vi "LibXML_AddNextSibling.vi"(8 "error in":errorcluster, 10 "sibling node":u32, 11 "new node":u32) -> (0 "error out":errorcluster, 3 "node copy":u32)   [LabVIEW 2019, in "Tools.lvlib" / "LibXML.lvlib"]
doc: "libXML2:\nFunction: xmlAddNextSibling\n\nxmlNodePtr xmlAddNextSibling (xmlNodePtr cur, xmlNodePtr elem)\n\n\nAdd a new node @elem as the next sibling of @cur If the new node was already inserted in \na document it is first unlinked from its existing context. As a result of text merging @elem\nmay be freed. If the new node is ATTRIBUTE, it is added into properties instead of children. \nIf there is an attribute with equal name, it is first destroyed.\n\nparent: the parent node\ncur: the child node\nReturns: the child or NULL in case of error."
uses:
  LibXML.lvlib
  dll/libxml2.dll
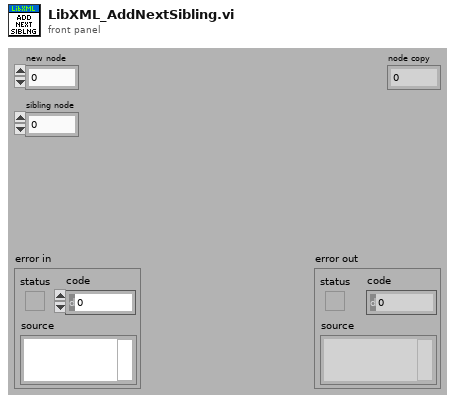
[diagram p1: front panel]
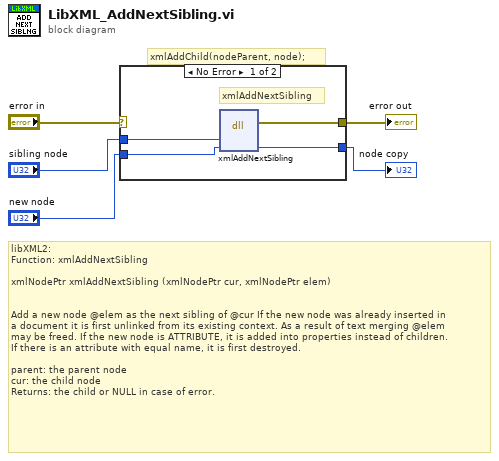
[diagram p0: block diagram]
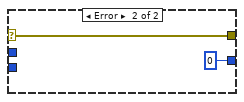
[diagram p2: hidden frame]
diagram:
  # "libXML2:\nFunction: xmlAddNextSibling\n\nxmlNodePtr\txmlAddNextSibling\t(xmlNodePtr cur, xmlNodePtr elem)\n\n\nAdd a new node @elem as the next sibling of @cur If the new node was already inserted in \na document it is first unlinked from its existing context. As a result of text merging @elem\nmay be freed. If the new node is ATTRIBUTE, it is added into properties instead of children. \nIf there is an attribute with equal name, it is first destroyed.\n\nparent:\tthe parent node\ncur:\tthe child node\nReturns:\tthe child or NULL in case of error."
  # "xmlAddChild(nodeParent, node);"
  n1 = case shown="No Error" "error in" {
    selector: "error in" -> [_ w11]
    tunnel: [w6 w11] -> w4
    tunnel: "new node" -> [w9 _]
    tunnel: "sibling node" -> [w8 _]
    tunnel: [w7 u32 0 ("node")] -> w1
    frame No Error {
      # "xmlAddNextSibling"
      n2 = dll-call lib="C:/Projects/_Prywatne/MyCIT/Framework/Tools/XML/LibXML/dll/libxml2.dll" fn="xmlAddNextSibling"("parent"=w8, "node"=w9) -> (error out=w6:errorcluster, "node"=w7:u32)  [unwired: 5 in, 1 out]
    }
    frame Error {
    }
  }
  "error out" <- w4
  "node copy" <- w1
